vi "Configuration(FGV).vi"(6 "File FGV Method":T1, 8 "error in":errorcluster, 11 "Configuration In":T2) -> (0 "error out":errorcluster, 3 "Configuration Out":T2)   [LabVIEW 2020, in "SECS Bridge.lvlib"]
uses:
  SECS Bridge.lvlib
  Configuration.ctl
  File FGV Method.ctl
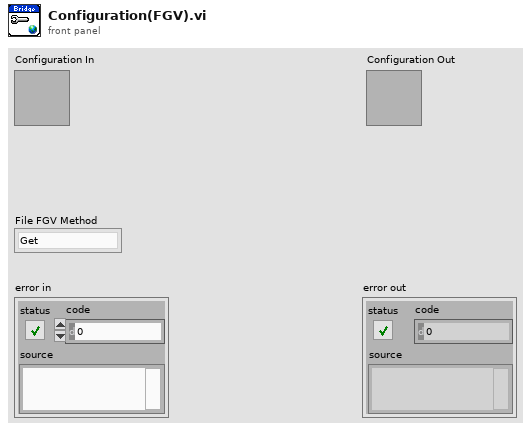
[diagram p1: front panel]
types:
  T1 = typedef "SECS Bridge.lvlib/File FGV Method.ctl" = enum16{"Get", "Put", "Read", "Write"}
  T2 = typedef "SECS Bridge.lvlib/Configuration.ctl" = cluster{"T3(Reply Timeout)":i32, "T5(Separation Timeout)":i32, "T6(Control Timeout)":i32, "T7(Not Selected Timeout)":i32, "T8(Inter-Character Timeout)":i32, "Session ID":u16, "Log Path":path, "IP Address":string, "Port":u16}
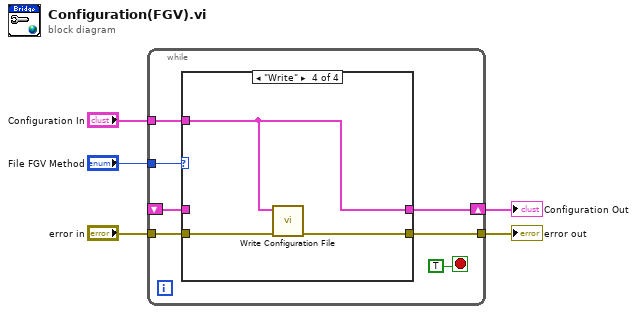
[diagram p0: block diagram]
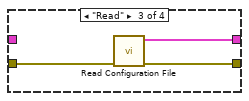
[diagram p4: hidden frame]
diagram:
  n1 = while {
    tunnel: "error in" -> [w12]
    tunnel: "File FGV Method" -> [w11]
    shift-right: [w10] -> w2
    shift-left: _ -> [w9]
    tunnel: "Configuration In" -> [w8]
    tunnel: [w7] -> w1
    stop <- TRUE stop-if-true
    n2 = case shown="\"Write\"" w11 {
      tunnel: w12 -> [w13 w15 w19 w22]
      tunnel: w9 -> [w14 _ _ _]
      tunnel: [w14 w16 w17 w20] -> w10
      tunnel: w8 -> [_ w16 _ w20]
      tunnel: [w13 w15 w18 w21] -> w7
      frame "Get", Default {
      }
      frame "Put" {
      }
      frame "Read" {
        n3 = call "Read Configuration File.vi"("error in"=w19) -> ("error out"=w18:errorcluster, "Configuration"=w17:T2)  [unwired: 9 in]
      }
      frame "Write" {
        n4 = call "Write Configuration File.vi"("error in"=w22, "Configuration"=w20) -> ("error out"=w21:errorcluster)  [unwired: 9 in]
      }
    }
  }
  "Configuration Out" <- w2
  "error out" <- w1
